vi "APS save param to file.vi"(8 "error in (no error)":errorcluster caption="错误输入（无错误）", 10 "pXMLFile":string, 11 "Board_ID":i32) -> (0 "error out":errorcluster caption="错误输出", 3 "function return":i32)   [LabVIEW 2011, in "APS168.lvlib"]
doc: "I32 FNTYPE APS_save_param_to_file( I32 Board_ID, const char *pXMLFile );"
uses:
  APS168.lvlib
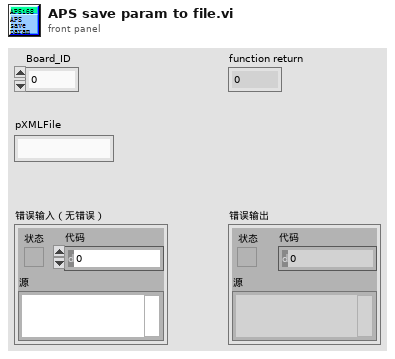
[diagram p1: front panel]
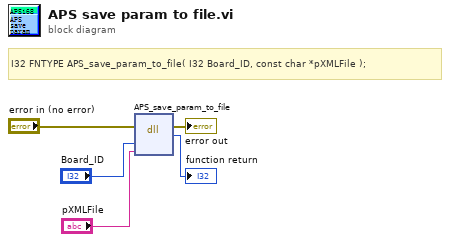
[diagram p0: block diagram]
diagram:
  # "I32 FNTYPE APS_save_param_to_file( I32 Board_ID, const char *pXMLFile );"
  n1 = dll-call lib="PTH1Labs E软件ADLINK 204CAPS_1_7_1_LIB line 连续运动204APS168.*" fn="APS_save_param_to_file"(error in="error in (no error)", "Board_ID"="Board_ID", "pXMLFile"="pXMLFile") -> (error out=→"error out":errorcluster, →"function return":i32)  [unwired: 4 in, 1 out]
